vi "BeltFeeder Controller.vi"(8 "error in":errorcluster) -> ()   [LabVIEW 2019]
doc: "This VI executes continuously carrying out the current operation and responding to updates or new operations. It will often contain the timing or control code that is difficult to place directly in TeleOp. This VI generally opens all sensors and motors and isolates the rest of the robot code from knowing how the operations are carried out."
uses:
  BeltFeeder Setpoints.ctl
  BeltFeeder Operations.ctl
  <vilib>/Rock Robotics/WPI/ThirdParty/Phoenix-LabVIEW/Motor Controller/Controls/CTRE_Phoenix_MotorControl_NeutralMode.ctl
  <vilib>/Rock Robotics/WPI/ThirdParty/Phoenix-LabVIEW/Motor Controller/Controls/CTRE_Phoenix_MotorControl_ControlMode.ctl
  <vilib>/Rock Robotics/Network Tables/NT Write Boolean.vi
panel:
  out "Current\nCmd":string
  # "Tip: It may be helpful to observe inputs and sensor values.\nYou may also want to display tuning or debugging controls."
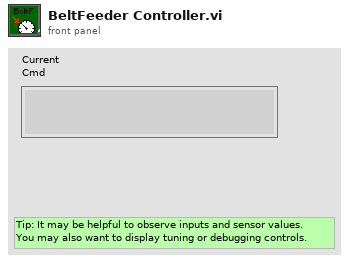
[diagram p1: front panel]
types:
  T1 = typedef "CTRE_Phoenix_MotorControl_ControlMode.ctl" = u16
  T2 = typedef "CTRE_Phoenix_MotorControl_NeutralMode.ctl" = enum8{"EEPROMSetting", "Override to Coast", "Override to Brake"}
  T3 = typedef "BeltFeeder Setpoints.ctl" = cluster{"Operation":T4, "Setpoint":dbl, "Duration":dbl}
  T4 = typedef "BeltFeeder Operations.ctl" = enum16{"Reserve", "Read Current", "Immediate", "Up", "Down", "Shoot"}
  T5 = typedef "WPI_MotorControlDeviceRef.ctl" = cluster{"DeviceStatus":errorcluster, "Type":T6, "PWM":cluster{"PWM Channel":T7, "DeadBand":T8}, "CAN":cluster{"Device Number":u8, "SetOutput VI Ref":variant, "GetOutput VI Ref":variant, "Enable VI Ref":variant, "Disable VI Ref":variant, "Data":variant}, "Invert":bool, "DIO PWM":cluster{"PWM \"Enable\" Channel":T7, "DIOChannel":T9, "PWM Rate":dbl}}
  T6 = typedef "WPI_MotorControlType.ctl" = enum16{"PWM", "CAN", "DIO PWM"}
  T7 = typedef "FPGA_DIOPWMChannel.ctl" = enum8{"PWM 0", "PWM 1", "PWM 2", "PWM 3", "PWM 4", "PWM 5", "PWM 6", "PWM 7", "PWM 8", "PWM 9", "PWM MXP 0", "PWM MXP 1", "PWM MXP 2", "PWM MXP 3", "PWM MXP 4", "PWM MXP 5", "PWM MXP 6", "PWM MXP 7", "PWM MXP 8", "PWM MXP 9", "Invalid"}
  T8 = typedef "WPI_PWMDeadband.ctl" = cluster{"Name":string, "maxPositivePwm":i32, "minPositivePwm":i32, "centerPwm":i32, "maxNegativePwm":i32, "minNegativePwm":i32, "angularRange":u16}
  T9 = typedef "FPGA_DIOChannel.ctl" = enum8{"DIO 0", "DIO 1", "DIO 2", "DIO 3", "DIO 4", "DIO 5", "DIO 6", "DIO 7", "DIO 8", "DIO 9", "DIO MXP 0", "DIO MXP 1", "DIO MXP 2", "DIO MXP 3", "DIO MXP 4", "DIO MXP 5", "DIO MXP 6", "DIO MXP 7", "DIO MXP 8", "DIO MXP 9", "DIO MXP 10", "DIO MXP 11", "DIO MXP 12", "DIO MXP 13", "DIO MXP 14", "DIO MXP 15", "SPI Port CS1", "SPI Port CS2", "SPI Port CS3", "SPI Port MISO", "SPI Port MOSI", "Invalid"}
  T10 = typedef "Command Status Info.ctl" = cluster{"Name":string, "Status":T11, "notifier out":T12}
  T11 = typedef "Completion Status.ctl" = enum16{"Successful", "Aborted", "Incomplete"}
  T12 = typedef "Completion Notifier.ctl" = refnum<notifier>
  T13 = cluster{"Current Command":T3, "Command Timing":cluster{"Start Time (ms)":u32, "Iterations":i32}, "Command Arguments":cluster{"Command Info":T10, "Description":string, "Default Command":T3, "queue out":refnum<queue>, "Subsystem Name":string}}
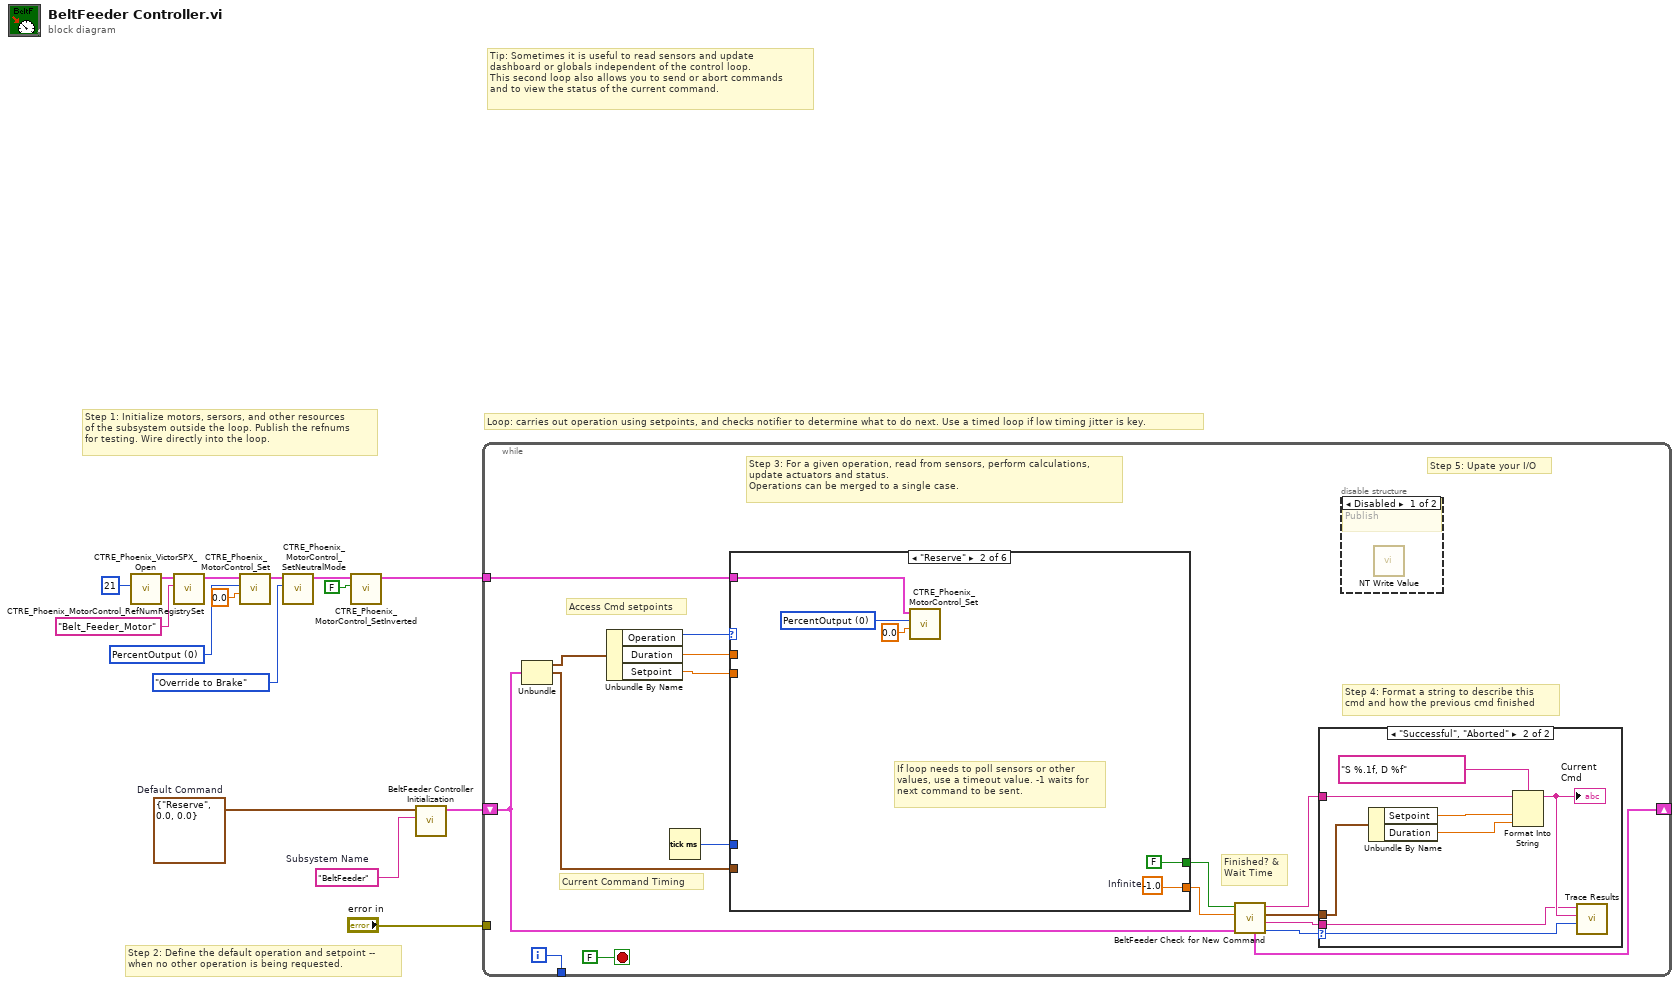
[diagram p0: block diagram]
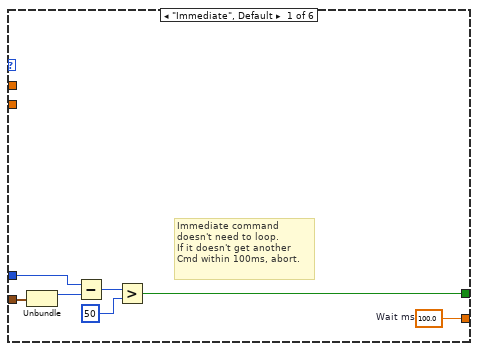
[diagram p4: hidden frame]
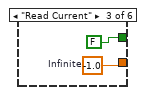
[diagram p5: hidden frame]
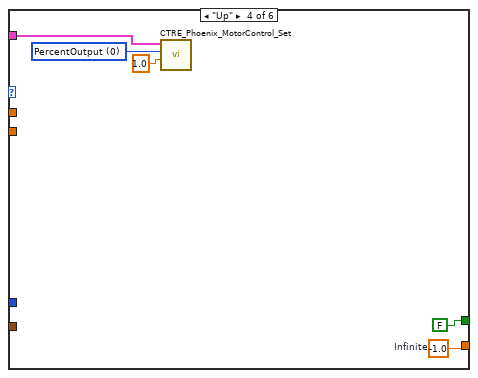
[diagram p6: hidden frame]
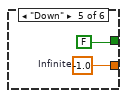
[diagram p7: hidden frame]
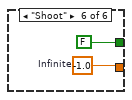
[diagram p8: hidden frame]
diagram:
  w3 = T1 0 items=["PercentOutput"=0, "Position"=1, "Velocity"=2, "Current"=3, "Follower"=5, "MotionProfile"=6, "MotionMagic"=7, "MotionProfileArc"=10, "Disabled"=15] ("Control Mode")
  w12 = T3 {"Operation"=enum."Reserve", "Setpoint"=0.0, "Duration"=0.0}  # Default Command
  w13 = "BeltFeeder"  # Subsystem Name
  # "Tip: Sometimes it is useful to read sensors and update\ndashboard or globals independent of the control loop.\nThis second loop also allows you to send or abort commands\nand to view the status of the current command."
  # "Step 2: Define the default operation and setpoint --\nwhen no other operation is being requested."
  # "Step 1: Initialize motors, sersors, and other resources\nof the subsystem outside the loop. Publish the refnums\nfor testing. Wire directly into the loop."
  # "Loop: carries out operation using setpoints, and checks notifier to determine what to do next. Use a timed loop if low timing jitter is key."
  n1 = call <vilib>:"CTRE_Phoenix_VictorSPX_Open.vi"("Device Number"=u8 21) -> ("CAN Talon SRX Ref"=w9:T5)  [unwired: 9 in, 1 out]
  n2 = call <vilib>:"CTRE_Phoenix_MotorControl_RefNumRegistrySet.vi"("refnum name"="Belt_Feeder_Motor", "PhoenixMotorControlDevRef"=w9) -> ("PhoenixMotorControlDevRef"=w10:T5)  [unwired: 8 in, 1 out]
  n3 = call <vilib>:"CTRE_Phoenix_MotorControl_Set.vi"("Output"=0.0, "Control Mode"=w3, "PhoenixMotorControlDevRef"=w10) -> ("PhoenixMotorControlDevRef"=w11:T5)  [unwired: 7 in, 1 out]
  n4 = call <vilib>:"CTRE_Phoenix_MotorControl_SetNeutralMode.vi"("Motor Control Neutral Mode"=CTRE_Phoenix_MotorControl_NeutralMode."Override to Brake", "PhoenixMotorControlDevRef"=w11) -> ("PhoenixMotorControlDevRef"=w6:T5)  [unwired: 8 in, 1 out]
  n5 = call <vilib>:"CTRE_Phoenix_MotorControl_SetInverted.vi"("Invert?"=FALSE, "PhoenixMotorControlDevRef"=w6) -> ("PhoenixMotorControlDevRef"=w1:T5)  [unwired: 8 in, 1 out]
  n6 = call "BeltFeeder Controller Initialization.vi"("Subsystem Name"=w13, "Default Command"=w12) -> ("Current Command"=w14:T13)  [unwired: 9 in]
  n7 = while {
    shift-right: [w24] -> _
    shift-left: w14 -> [w17]
    tunnel: [w31] -> _
    tunnel: "error in" -> [_]
    tunnel: w1 -> [w16]
    i -> [w31]
    stop <- FALSE stop-if-true
    # "Step 5: Upate your I/O"
    # "Step 4: Format a string to describe this\ncmd and how the previous cmd finished"
    # "Current Command Timing"
    # "Access Cmd setpoints"
    # "Finished? &\nWait Time"
    # "Step 3: For a given operation, read from sensors, perform calculations,\nupdate actuators and status.\nOperations can be merged to a single case."
    n8 = Unbundle(w17) -> ("Current Command"=w30:T3, "Command Timing"=w26:cluster{"Start Time (ms)":u32, "Iterations":i32})  [unwired: 1 out]
    n9 = Unbundle By Name(w30) -> ("Operation"=w29:T4, "Duration"=w28:dbl, "Setpoint"=w25:dbl)
    n10 = Tick Count (ms)() -> (millisecond timer value=w27:u32)
    n11 = case shown="\"Reserve\"" w29 {
      tunnel: [w47 w52 w53 w58 w60 w62] -> w22
      tunnel: [w41 FALSE ("ignore previous (F)") FALSE ("ignore previous (F)") FALSE ("ignore previous (F)") FALSE ("ignore previous (F)") FALSE ("ignore previous (F)")] -> w23
      tunnel: w26 -> [w43 _ _ _ _ _]
      tunnel: w28 -> [_ _ _ _ _ _]
      tunnel: w27 -> [w42 _ _ _ _ _]
      tunnel: w25 -> [_ _ _ _ _ _]
      tunnel: w16 -> [_ w48 _ w57 _ _]
      frame "Immediate", Default {
        w47 = 100.0  # Wait ms
        # "Immediate command\ndoesn't need to loop.\nIf it doesn't get another\nCmd within 100ms, abort."
        n12 = Unbundle(w43) -> ("Start Time (ms)"=w46:u32)  [unwired: 1 out]
        n13 = Subtract(x=w42, y=w46) -> (x-y=w45:u32)
        n14 = Greater?(x=w45, y=u8 50 ("Left Motor")) -> (0:w41:bool)
      }
      frame "Reserve" {
        w50 = T1 0 items=["PercentOutput"=0, "Position"=1, "Velocity"=2, "Current"=3, "Follower"=5, "MotionProfile"=6, "MotionMagic"=7, "MotionProfileArc"=10, "Disabled"=15] ("Control Mode")
        w52 = -1.0  # Infinite
        # "If loop needs to poll sensors or other\nvalues, use a timeout value. -1 waits for\nnext command to be sent."
        n15 = call <vilib>:"CTRE_Phoenix_MotorControl_Set.vi"("Output"=0.0, "Control Mode"=w50, "PhoenixMotorControlDevRef"=w48) -> ()  [unwired: 7 in, 2 out]
      }
      frame "Read Current" {
        w53 = -1.0  # Infinite
      }
      frame "Up" {
        w56 = T1 0 items=["PercentOutput"=0, "Position"=1, "Velocity"=2, "Current"=3, "Follower"=5, "MotionProfile"=6, "MotionMagic"=7, "MotionProfileArc"=10, "Disabled"=15] ("Control Mode")
        w58 = -1.0  # Infinite
        n16 = call <vilib>:"CTRE_Phoenix_MotorControl_Set.vi"("Output"=1.0, "Control Mode"=w56, "PhoenixMotorControlDevRef"=w57) -> ()  [unwired: 7 in, 2 out]
      }
      frame "Down" {
        w60 = -1.0  # Infinite
      }
      frame "Shoot" {
        w62 = -1.0  # Infinite
      }
    }
    n17 = call "BeltFeeder Check for New Command.vi"("Current Command"=w17, "Wait time (ms)"=w22, "Finished?"=w23) -> ("Completion"=w18:T11, "Subsystem Name"=w19:string, "Current Command"=w20:T3, "Initial Trace String"=w21:string, "NextCommand"=w24:T13)  [unwired: 4 in]
    n18 = case shown="\"Successful\", \"Aborted\"" w18 {
      selector: w18 -> [_ w40]
      tunnel: w21 -> [_ w36]
      tunnel: w20 -> [_ w37]
      tunnel: w19 -> [_ w33]
      frame "Incomplete", Default {
        # "Continuing current command"
      }
      frame "Successful", "Aborted" {
        # "Report and setup for next command"
        n19 = Unbundle By Name(w37) -> ("Setpoint"=w39:dbl, "Duration"=w34:dbl)
        n20 = Format Into String(format string="S %.1f, D %f", initial string=w36, w39, w34) -> (resulting string=w35:string)  [unwired: 1 in, 1 out]
        "Current\nCmd" <- w35
        n21 = call <vilib>:"Trace Results.vi"("Status of previous command"=w40, "Description"=w35, "Subsystem"=w33) -> ()  [unwired: 9 in]
      }
    }
    n22 = disable-structure shown="Disabled" {
      frame Disabled {
        # "Publish"
        n23 = call-poly <vilib>:"NT Write Value.vi"() -> ()  [unwired: 11 in, 1 out]
      }
      frame Enabled {
      }
    }
  }
